vi "Read Session Valid.vi"(8 "error in (no error)":errorcluster, 11 "MB_Master in":refnum<class "MB_Master.lvclass">) -> (0 "error out":errorcluster, 2 "Valid?":bool, 3 "MB_Master out":refnum<class "MB_Master.lvclass">)   [LabVIEW 2016, in "MB Master.lvlib" / "MB_Master.lvclass"]
uses:
  MB_Master.lvclass
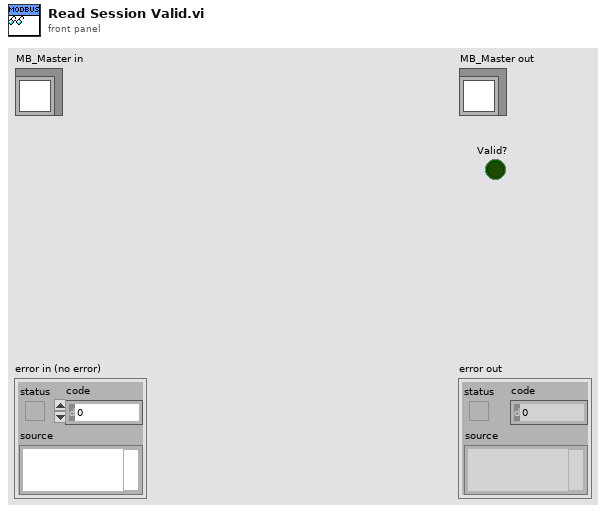
[diagram p1: front panel]
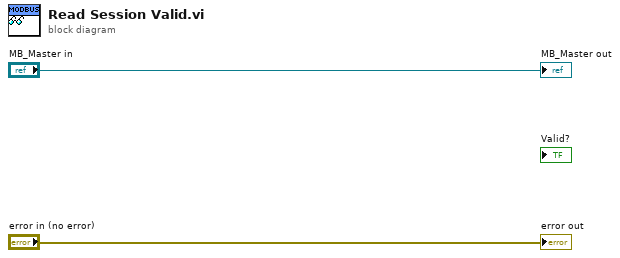
[diagram p0: block diagram]
diagram:
  "error out" <- "error in (no error)"
  "MB_Master out" <- "MB_Master in"
